vi "F Dwf Digital Spi Read One.vi"(7 "pRX":u32, 8 "error in (no error)":errorcluster, 9 "cBitPerWord":i32, 10 "cDQ":i32, 11 "hdwf":i32) -> (0 "error out":errorcluster, 3 "function return":i32, 5 "pRX out":u32)   [LabVIEW 2021, in "Olasdwf.lvlib"]
doc: "DWFAPI int FDwfDigitalSpiReadOne(HDWF hdwf, int cDQ, int cBitPerWord, unsigned int *pRX);"
uses:
  Olasdwf.lvlib
  Windows/System32/dwf.dll
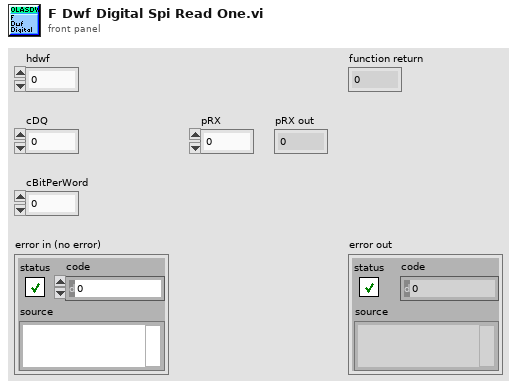
[diagram p1: front panel]
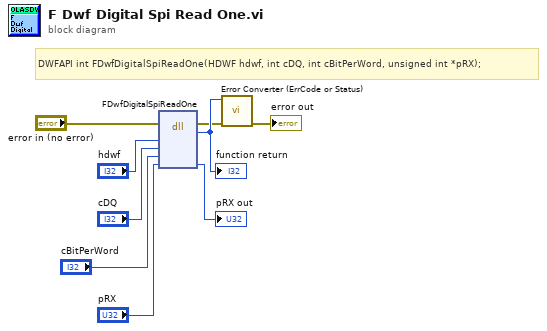
[diagram p0: block diagram]
diagram:
  # "DWFAPI int FDwfDigitalSpiReadOne(HDWF hdwf, int cDQ, int cBitPerWord, unsigned int *pRX);"
  n1 = dll-call lib="/Windows/System32/dwf.*" fn="FDwfDigitalSpiReadOne"(error in="error in (no error)", "hdwf"="hdwf", "cDQ"="cDQ", "cBitPerWord"="cBitPerWord", "pRX"="pRX") -> (error out=w2:errorcluster, w9:i32, "pRX"=→"pRX out":u32)  [unwired: 5 in, 1 out]
  "function return" <- w9
  n2 = call "Error Converter (ErrCode or Status).vi"("error in (no error)"=w2, "error code"=w9) -> ("error out"=→"error out":errorcluster)  [unwired: 9 in]
